vi "dfd_Generate Quantized Coefficients Report.vi"(5 "structure type":T1, 7 "quant settings":T2={"source"=0, "wl"=1, "iwl"=0, "overflow mode"=enum."Saturation", "rounding mode"=enum."Nearest", "signed?"=TRUE} {"source" items=["Coef a/k"=0, "Coef b/v"=7, "Input"=1, "Output"=2, "Multiplicand"=3, "Product"=4, "Sum"=5, "Delay"=6, "Gain"=8]}, 8 "error in (no error)":errorcluster, 9 "prefix":string, 10 "quantized coef":dbl[](array[numeric]) format="%.2f", 11 "reference coef":dbl[](array[numeric]) format="%.2f") -> (0 "error out":errorcluster, 3 "report":string)   [LabVIEW 2017, in "NI_DigFilter_FXP.lvlib"]
uses:
  <vilib>/addons/Digital Filter Design/NI_DigFilter_FXP.lvlib
  <vilib>/addons/Digital Filter Design/_Objects.llb/dfd_Internal Quantization Settings.ctl
  <vilib>/addons/Digital Filter Design/_Objects.llb/dfd_Internal Quantization Srcs.ctl
  <vilib>/addons/Digital Filter Design/_Objects.llb/DFD Filter Structure Type Selector.ctl
  <vilib>/addons/Digital Filter Design/NI_DigFilterLicensed.lvlib
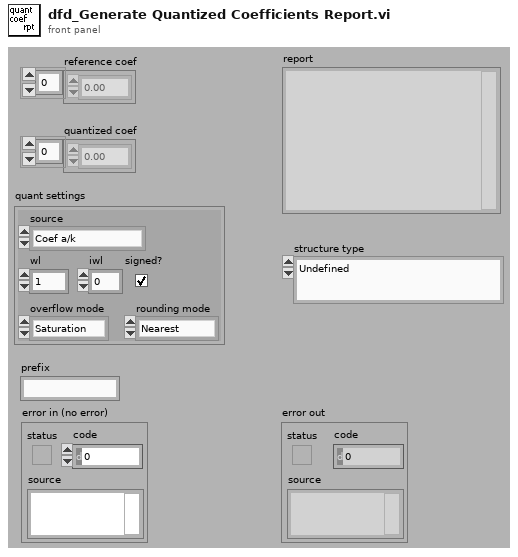
[diagram p1: front panel]
types:
  T1 = typedef "NI_DigFilterLicensed.lvlib/DFD Filter Structure Type Selector.ctl" = enum16{"Undefined", "FIR Direct Form", "FIR Direct Form Transposed", "FIR Symmetric", "FIR Antisymmetric", "IIR Direct Form I", "IIR Direct Form I Transposed", "IIR Direct Form II", "IIR Direct Form II Transposed", "IIR Cascaded Second Order Sections Form I", "IIR Cascaded Second Order Sections Form I Transposed", "IIR Cascaded Second Order Sections Form II", "IIR Cascaded Second Order Sections Form II Transposed", "Lattice Allpass (basic sections)", "Lattice Allpass (one multiplier sections)", "Lattice Allpass (normalized sections)", "Lattice AR (basic sections)", "Lattice AR (one multiplier sections)", "Lattice AR (normalized sections)", "Lattice MA (minimum phase)", "Lattice MA (maximum phase)", "Lattice ARMA (basic sections)", "Lattice ARMA (one multiplier sections)", "Lattice ARMA (normalized sections)"}
  T2 = typedef "NI_DigFilterLicensed.lvlib/dfd_Internal Quantization Settings.ctl" = cluster{"source":T3, "wl":i16, "iwl":i16, "overflow mode":enum16{"Saturation", "Wrap"}, "rounding mode":enum16{"Nearest", "Truncation"}, "signed?":bool}
  T3 = typedef "NI_DigFilterLicensed.lvlib/dfd_Internal Quantization Srcs.ctl" = u16
  T4 = typedef "NI_DigFilterLicensed.lvlib/DFD Filter Structure Id.ctl" = enum16{"Undefined", "FIR", "IIR Direct", "IIR SOS", "IIR Allpass", "IIR AR", "IIR ARMA"}
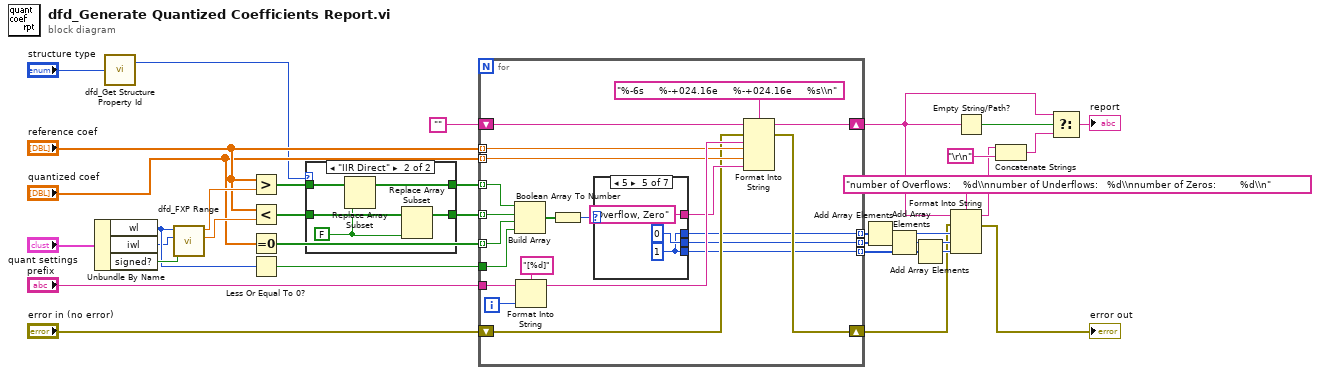
[diagram p0: block diagram]
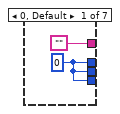
[diagram p3: hidden frame]
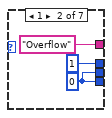
[diagram p4: hidden frame]
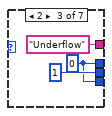
[diagram p5: hidden frame]
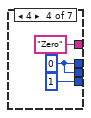
[diagram p6: hidden frame]
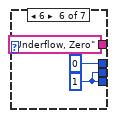
[diagram p7: hidden frame]
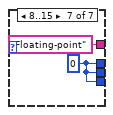
[diagram p8: hidden frame]
diagram:
  n1 = Unbundle By Name("quant settings") -> ("wl"=w2:i16, "iwl"=w1:i16, "signed?"=w30:bool)
  n2 = call <vilib>:"dfd_Get Structure Property Id.vi"("structure type"="structure type") -> ("filter structure id"=w7:T4)  [unwired: 1 out]
  n3 = call <vilib>:"dfd_FXP Range.vi"("signed?"=w30, "iwl"=w1, "wl"=w2) -> ("low"=w32:ext, "high"=w31:ext)  [unwired: 7 out]
  n4 = Greater?(x="reference coef", y=w31) -> (0:w6:bool[])
  n5 = Less?(x="reference coef", y=w32) -> (x < y?=w5:bool[])
  n6 = Equal To 0?(x="quantized coef") -> (x = 0?=w34:bool[])
  n7 = Less Or Equal To 0?(x=w2) -> (x <= 0?=w11:bool)
  n8 = case shown="\"IIR Direct\"" w7 {
    tunnel: w6 -> [w36 w41]
    tunnel: w5 -> [w35 w40]
    tunnel: [w36 w38] -> w4
    tunnel: [w35 w37] -> w3
    frame "Undefined", Default {
    }
    frame "IIR Direct" {
      w39 = FALSE
      n9 = Replace Array Subset(array=w41, new element=w39) -> (w38:bool[])  [unwired: 1 in]
      n10 = Replace Array Subset(array=w40, new element=w39) -> (w37:bool[])  [unwired: 1 in]
    }
  }
  n11 = for {
    tunnel: "reference coef" -> [w56] mode=indexing
    tunnel: "quantized coef" -> [w55] mode=indexing
    shift-right: [w60] -> w16
    shift-left: "" -> [w61]
    tunnel: w4 -> [w52] mode=indexing
    tunnel: w3 -> [w53] mode=indexing
    tunnel: "prefix" -> [w54]
    tunnel: w34 -> [w51] mode=indexing
    shift-right: [w46] -> w19
    shift-left: "error in (no error)" -> [w47]
    tunnel: [w45] -> w26 mode=indexing
    tunnel: [w44] -> w25 mode=indexing
    tunnel: [w43] -> w24 mode=indexing
    tunnel: w11 -> [w42]
    i -> [w59]
    n12 = Build Array(w52, w53, w51, w42) -> (w50:bool[])
    n13 = Format Into String(format string="[%d]", initial string=w54, w59) -> (resulting string=w57:string)  [unwired: 1 in, 1 out]
    n14 = Boolean Array To Number(Boolean array=w50) -> (number=w49:u32)
    n15 = case shown="5" w49 {
      tunnel: ["" "Overflow" "Underflow" "Zero" "Overflow, Zero" "Underflow, Zero" "Floating-point"] -> w48
      tunnel: [w63 1 w68 w71 w74 0 w80] -> w45
      tunnel: [w63 w65 1 w71 0 w77 w80] -> w44
      tunnel: [w63 w65 w68 1 w74 w77 w80] -> w43
      frame 0, Default {
        w63 = 0
      }
      frame 1 {
        w65 = 0
      }
      frame 2 {
        w68 = 0
      }
      frame 4 {
        w71 = 0
      }
      frame 5 {
        w74 = 1
      }
      frame 6 {
        w77 = 1
      }
      frame 8..15 {
        w80 = 0
      }
    }
    n16 = Format Into String(format string="%-6s     %-+024.16e     %-+024.16e     %s\\n", initial string=w61, error in=w47, w57, w56, w55, w48) -> (resulting string=w60:string, error out=w46:errorcluster)
  }
  n17 = Add Array Elements(numeric array=w26) -> (sum=w22:i32)
  n18 = Add Array Elements(numeric array=w25) -> (sum=w21:i32)
  n19 = Add Array Elements(numeric array=w24) -> (sum=w20:i32)
  n20 = Format Into String(format string="number of Overflows:    %d\\nnumber of Underflows:   %d\\nnumber of Zeros:        %d\\n", initial string=w16, error in=w19, w22, w21, w20) -> (resulting string=w13:string, error out=→"error out":errorcluster)
  n21 = Empty String/Path?(string/path=w16) -> (empty?=w17:bool)
  n22 = Concatenate Strings(w13, "\r\n") -> (w12:string)
  n23 = Select(t=w16, s=w17, f=w12) -> (s? t:f=→"report":string)
